vi "gmmregRegistrationTestLowLevel.vi"() -> ()   [LabVIEW 2017]
uses:
  <vilib>/Utility/file.llb/Read Delimited Spreadsheet (DBL).vi
panel:
  out "x/y":dbl
  out "XY Graph 2":cluster{dbl[], dbl[]}[](graph)
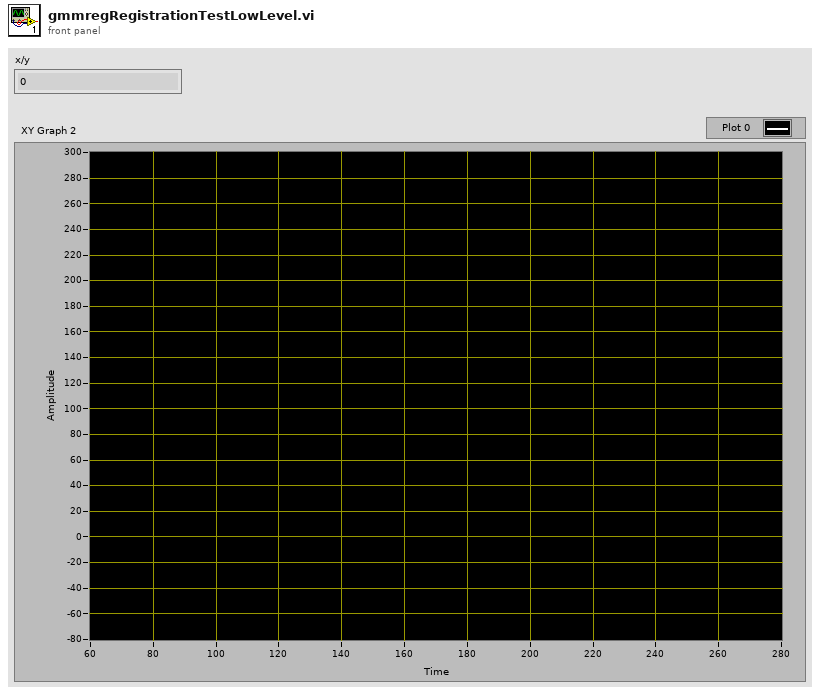
[diagram p1: front panel]
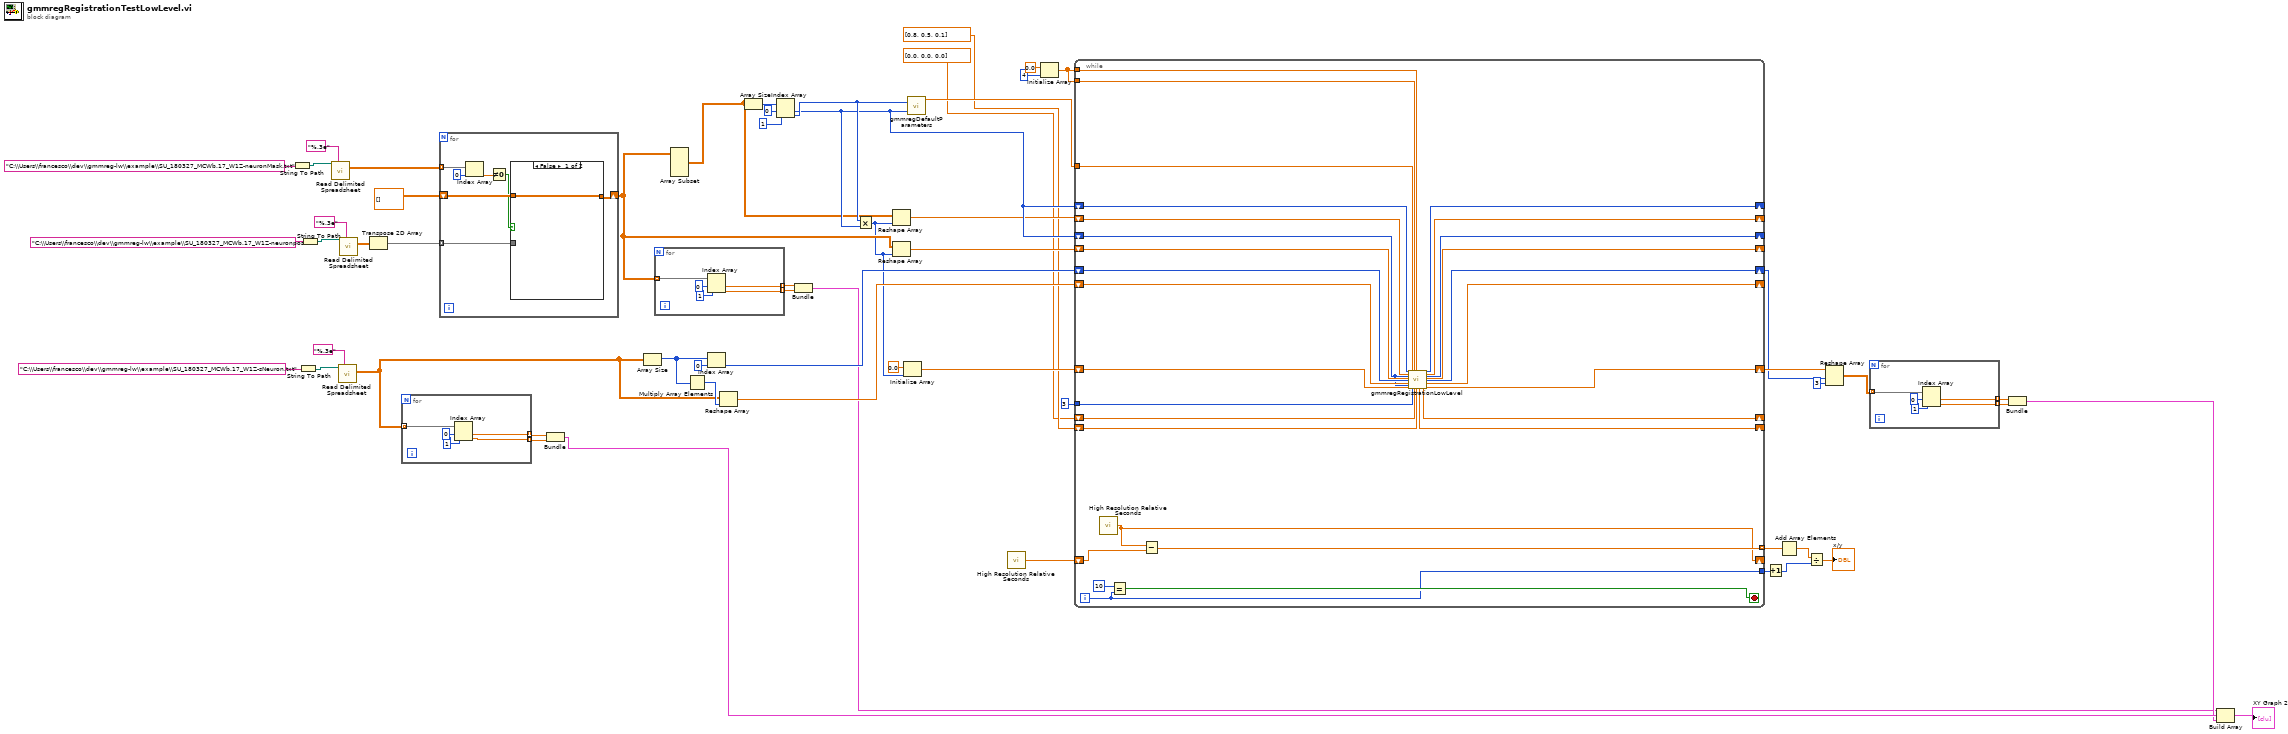
[diagram p0: block diagram]
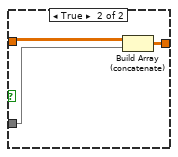
[diagram p2: hidden frame]
diagram:
  n1 = String To Path(string="C:\\Users\\francesco\\dev\\gmmreg-lw\\example\\SU_180327_MCWb.17_W1Z-neuronMask.txt") -> (path=w50:path)
  n2 = String To Path(string="C:\\Users\\francesco\\dev\\gmmreg-lw\\example\\SU_180327_MCWb.17_W1Z-sNeuron.txt") -> (path=w53:path)
  n3 = String To Path(string="C:\\Users\\francesco\\dev\\gmmreg-lw\\example\\SU_180327_MCWb.17_W1Z-neuronpos") -> (path=w57:path)
  n4 = call-poly <vilib>:"Read Delimited Spreadsheet.vi"("file path (dialog if empty)"=w50, "format (%.3f)"="%.3e") -> ("all rows"=w47:dbl[][])  [unwired: 8 in, 5 out]
  n5 = call-poly <vilib>:"Read Delimited Spreadsheet.vi"("file path (dialog if empty)"=w53, "format (%.3f)"="%.3e") -> ("all rows"=w32:dbl[][])  [unwired: 8 in, 5 out]
  n6 = call-poly <vilib>:"Read Delimited Spreadsheet.vi"("file path (dialog if empty)"=w57, "format (%.3f)"="%.3e") -> ("all rows"=w55:dbl[][])  [unwired: 8 in, 5 out]
  n7 = Transpose 2D Array(2D array=w55) -> (transposed array=w48:dbl[][])
  n8 = for {
    tunnel: w32 -> [w63] mode=indexing
    tunnel: [w60] -> w11 mode=indexing
    tunnel: [w59] -> w10 mode=indexing
    n9 = Index Array(array=w63, index #1=0 ("index"), index #2=1 ("index")) -> (element #1=w60:dbl, element #2=w59:dbl)
  }
  n10 = for {
    tunnel: w48 -> [w65] mode=indexing
    tunnel: w47 -> [w70] mode=indexing
    shift-right: [w64] -> w37
    shift-left: dbl[][] [] -> [w67]
    n11 = Index Array(array=w70, index=0) -> (element=w68:dbl)
    n12 = Not Equal To 0?(x=w68) -> (x != 0?=w66:bool)
    n13 = case shown="False" w66 {
      tunnel: w67 -> [w71 w74]
      tunnel: w65 -> [_ w73]
      tunnel: [w71 w72] -> w64
      frame False {
      }
      frame True {
        n14 = Build Array (concatenate)(w74, w73) -> (w72:dbl[][])
      }
    }
  }
  n15 = Bundle(w11, w10) -> (w9:cluster{dbl[], dbl[]})  [unwired: 1 in]
  n16 = Array Size(array=w32) -> (size(s)=w34:i32[])
  n17 = for {
    tunnel: w37 -> [w79] mode=indexing
    tunnel: [w76] -> w5 mode=indexing
    tunnel: [w75] -> w4 mode=indexing
    n18 = Index Array(array=w79, index #1=0 ("index"), index #2=1 ("index")) -> (element #1=w76:dbl, element #2=w75:dbl)
  }
  n19 = Array Subset(array=w37) -> (w39:dbl[][])  [unwired: 4 in]
  n20 = Multiply Array Elements(1:w34) -> (0:w33:i32)
  n21 = Index Array(array=w34, index=0) -> (element=w31:i32)
  n22 = Reshape Array(w32, w33) -> (w30:dbl[])
  n23 = Array Size(array=w39) -> (size(s)=w45:i32[])
  n24 = Index Array(array=w45, index #1=0 ("index"), index #2=1 ("index")) -> (element #1=w40:i32, element #2=w41:i32)
  n25 = Bundle(w5, w4) -> (w3:cluster{dbl[], dbl[]})  [unwired: 1 in]
  n26 = Multiply(x=w41, y=w40) -> (x*y=w28:i32)
  n27 = Reshape Array(w39, w28) -> (w38:dbl[])
  n28 = Reshape Array(w37, w28) -> (w36:dbl[])
  n29 = Initialize Array(0.0 ("element"), w28) -> (w27:dbl[])
  n30 = call "gmmregDefaultParameters.vi"("D (3)"=w41, "nctrlPts"=w40) -> ("param0"=w42:dbl[])  [unwired: 3 out]
  n31 = call <vilib>:"High Resolution Relative Seconds.vi"() -> ("relative seconds"=w22:dbl)
  n32 = Initialize Array(0.0 ("element"), 4 ("dimension size")) -> (w23:dbl[])
  n33 = while {
    shift-right: [w104] -> _
    shift-left: dbl[] [0.8, 0.5, 0.1] -> [w106]
    shift-right: [w103] -> _
    shift-left: dbl[] [0.0, 0.0, 0.0] -> [w105]
    shift-right: [w100] -> _
    shift-left: w40 -> [w102]
    shift-right: [w99] -> _
    shift-left: w38 -> [w101]
    shift-right: [w98] -> _
    shift-left: w40 -> [w92]
    shift-right: [w97] -> _
    shift-left: w36 -> [w96]
    shift-right: [w87] -> _
    shift-left: w30 -> [w95]
    shift-right: [w88] -> w15
    shift-left: w31 -> [w93]
    shift-right: [w86] -> w16
    shift-left: w27 -> [w94]
    tunnel: 3 -> [w91]
    tunnel: w42 -> [w107]
    tunnel: w23 -> [w90]
    tunnel: w23 -> [w89]
    shift-right: [w81] -> _
    shift-left: w22 -> [w83]
    tunnel: [w82] -> w20 mode=indexing
    tunnel: [w80] -> w21
    i -> [w80]
    stop <- w84 stop-if-true
    n34 = call <vilib>:"High Resolution Relative Seconds.vi"() -> ("relative seconds"=w81:dbl)
    n35 = Equal?(x=10, y=w80) -> (x = y?=w84:bool)
    n36 = Subtract(x=w81, y=w83) -> (x-y=w82:dbl)
    n37 = call "gmmregRegistrationLowLevel.vi"("nctrlpts"=w102, "coordCtrlPts"=w101, "npts"=w92, "coord"=w96, "nptsScene"=w93, "coordScene"=w95, "nOut"=w92, "out"=w94, "param0"=w107, "dim (3)"=w91, "normParams"=w89, "lambda"=w105, "denormParams"=w90, "scale"=w106) -> ("scale out"=w104:dbl[], "lambda out"=w103:dbl[], "nctrlpts out"=w100:i32, "coordCtrlPts out"=w99:dbl[], "npts out"=w98:i32, "coord out"=w97:dbl[], "nptsScene out"=w88:i32, "coordScene out"=w87:dbl[], "out out"=w86:dbl[])  [unwired: 5 out]
  }
  n38 = Increment(x=w21) -> (x+1=w18:i32)
  n39 = Add Array Elements(numeric array=w20) -> (sum=w19:dbl)
  n40 = Divide(x=w19, y=w18) -> (x/y=→"x/y":dbl)
  n41 = Reshape Array(w16, w15, 3 ("dimension size")) -> (w13:dbl[][])
  n42 = for {
    tunnel: w13 -> [w112] mode=indexing
    tunnel: [w109] -> w8 mode=indexing
    tunnel: [w108] -> w7 mode=indexing
    n43 = Index Array(array=w112, index #1=0 ("index"), index #2=1 ("index")) -> (element #1=w109:dbl, element #2=w108:dbl)
  }
  n44 = Bundle(w8, w7) -> (w6:cluster{dbl[], dbl[]})  [unwired: 1 in]
  n45 = Build Array(w3, w9, w6) -> (→"XY Graph 2":cluster{dbl[], dbl[]}[])
